vi "create.vi"(8 "error in":errorcluster) -> (0 "error out":errorcluster)   [LabVIEW 2020, in "main.lvlib" / "stopwatch_timer.lvlib"]
uses:
  stopwatch_timer.lvlib
  library_variable.vi
panel:
  # "Development\ncontrols/indicators useful for development and testing, but which are not outputs of the VI"
  # "Input\nInputs to the VI"
  # "Output\nOutputs of the VI"
  # "Description\n\nBlank VI with error handling case. \n\nSummarize the use of this VI in this space."
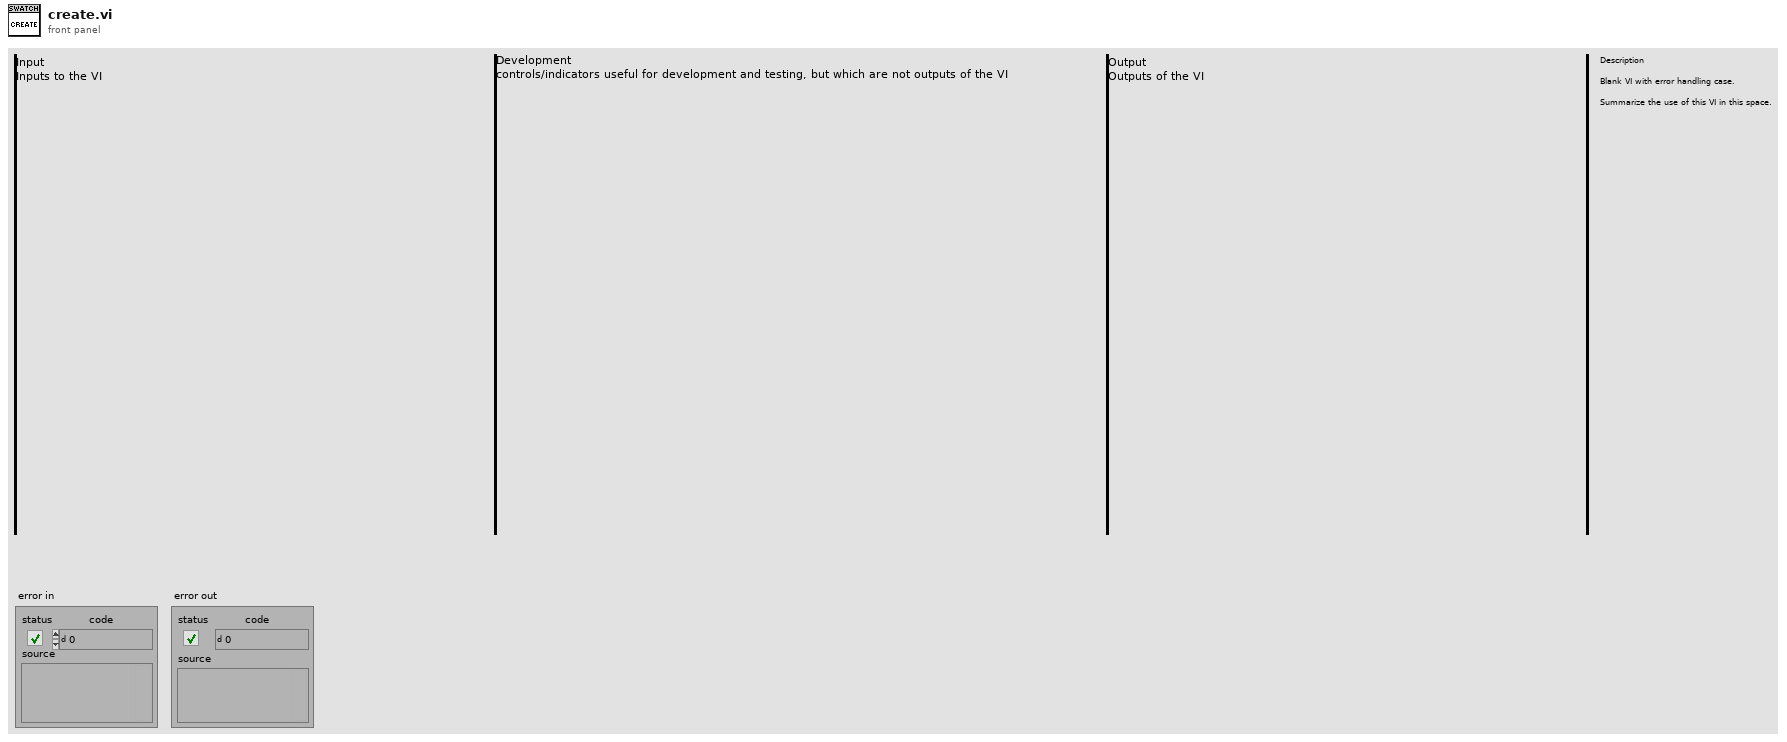
[diagram p1: front panel]
types:
  T1 = typedef "main.lvlib/stopwatch_timer.lvlib/stopwatch data.ctl" = cluster{"state":T2, "started at":timestamp, "last resumed at":timestamp, "last paused at":timestamp, "total time running (seconds)":dbl, "total time paused (seconds)":dbl}
  T2 = typedef "main.lvlib/stopwatch_timer.lvlib/state.ctl" = enum16{"not started", "running", "paused"}
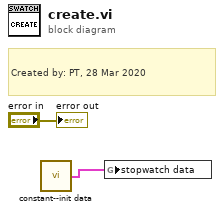
[diagram p0: block diagram]
diagram:
  # "Created by: PT, 28 Mar 2020"
  n1 = call "constant--init data.vi"() -> ("init data"=w1:T1)
  n2 = global write "library_variable.vi" "stopwatch data"(w1) -> ()
  "error out" <- "error in"
